vi "Centauro Verify Display Dryer.vi"(0 "GEA2 Reference In":refnum<k24>, 1 "Service Mode?":bool, 5 "UI GEA Inputs":T3={"Source"=228, "Destination"=37} {"Destination" format="%.0x"; "Source" format="%.0x"}, 7 "Care":T4={"Damp"=TRUE, "Dry"=TRUE, "Cool"=TRUE, "Eco"=TRUE}, 9 "Expected LED Status":T6, 11 "Error In":errorcluster, 12 "Erd_UiLedBitmap ERD #":T1[](array[typedef])=[{"ERD Number"=61729, "Data Type"=enum."string"}] {"ERD Number" format="%.0x"}, 13 "Erd_UiBlinkingLedBitmap ERD #":T1[](array[typedef])=[{"ERD Number"=61730, "Data Type"=enum."string"}] {"ERD Number" format="%.0x"}) -> (3 "Normal LED Binary Number Out":u32, 4 "GEA2 Reference Out":refnum<k24>, 6 "Pass/Fail?":bool, 8 "Report Text":string, 14 "Blinking LED Binary Number Out":u32, 15 "Error Out":errorcluster)   [LabVIEW 2016]
uses:
  Q:/Common/DLLs/GEA3/GeaCommunication.dll
  Common/DLLs/GEA3/GeaCommunication.dll
  Centauro Washer/Product Testcode/Centauro/Valew Common/type defs/LED Status OOB.ctl
  Common/LabVIEW GEA2 Toolkit/LabVIEW_GEA2_Toolkit.lvlibp/type defs/Source_Destination.ctl
  Common/LabVIEW GEA2 Toolkit/LabVIEW_GEA2_Toolkit.lvlibp/type defs/ERD Read Data In.ctl
  Common/LabVIEW GEA2 Toolkit/LabVIEW_GEA2_Toolkit.lvlibp/type defs/Data Type.ctl
  Common/LabVIEW GEA2 Toolkit/LabVIEW_GEA2_Toolkit.lvlibp
panel:
  in  "Board Index":i32
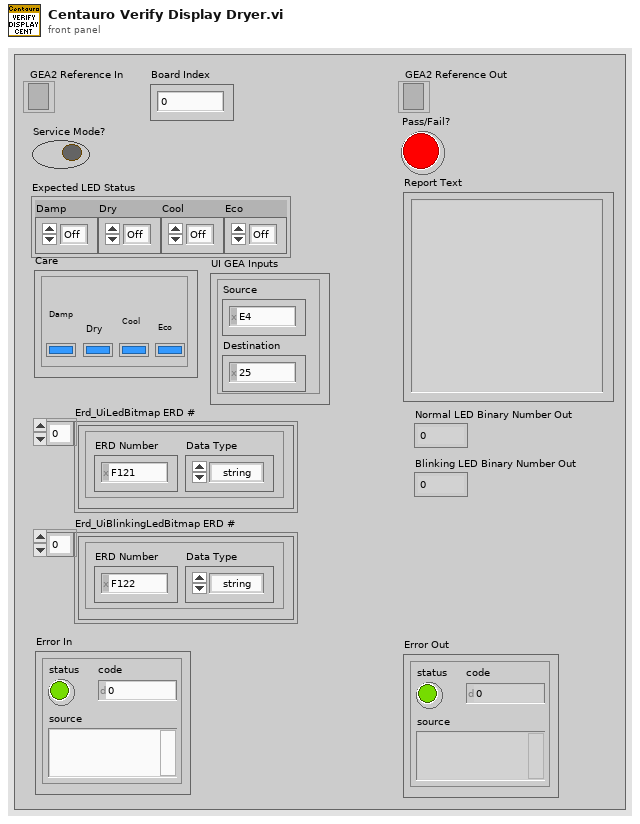
[diagram p1: front panel]
types:
  T1 = typedef "LabVIEW_GEA2_Toolkit.lvlibp/ERD Read Data In.ctl" = cluster{"ERD Number":u16, "Data Type":T2}
  T2 = typedef "LabVIEW_GEA2_Toolkit.lvlibp/Data Type.ctl" = enum16{"string", "boolean", "uint8_t", "uint16_t", "uint32_t", "uint64_t", "int8_t", "int16_t", "int32_t", "int64_t"}
  T3 = typedef "LabVIEW_GEA2_Toolkit.lvlibp/Source_Destination.ctl" = cluster{"Source":u8, "Destination":u8}
  T4 = cluster{"Damp":bool, "Dry":bool, "Cool":bool, "Eco":bool}
  T5 = typedef "LED Status OOB.ctl" = enum32{"Off", "On", "Blink"}
  T6 = cluster{"Damp":T5, "Dry":T5, "Cool":T5, "Eco":T5}
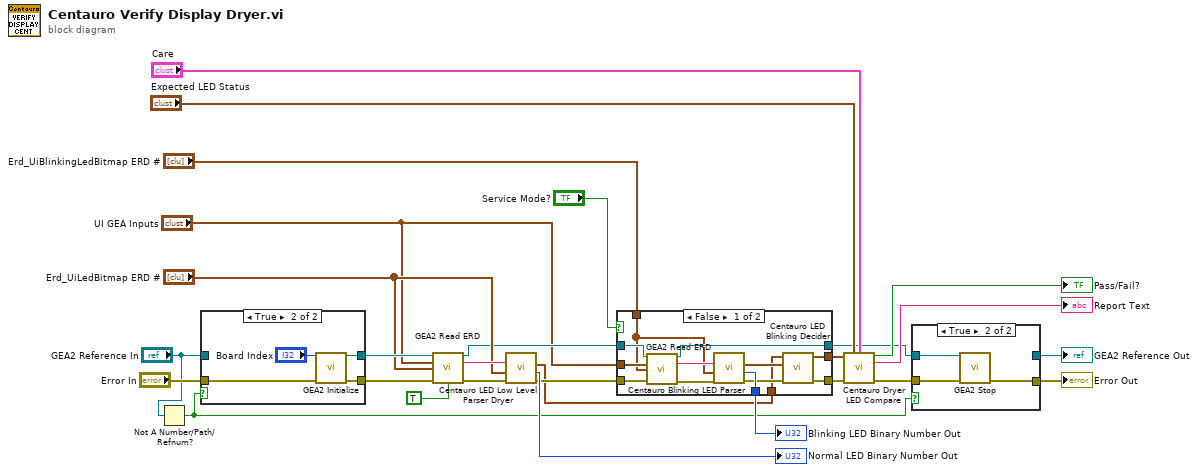
[diagram p0: block diagram]
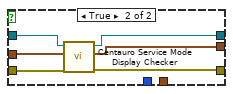
[diagram p2: hidden frame]
diagram:
  n1 = Not A Number/Path/Refnum?(number/path/refnum="GEA2 Reference In") -> (NaN/Path/Refnum?=w2:bool)
  n2 = case shown="True" w2 {
    tunnel: [w28 w33] -> w26
    tunnel: "Error In" -> [w28 w32]
    tunnel: [w29 w31] -> w24
    tunnel: "GEA2 Reference In" -> [w29 _]
    frame False {
    }
    frame True {
      n3 = call "GEA2 Initialize.vi"("Board Index"="Board Index", "error in"=w32) -> ("GEA2 Reference Out"=w31:refnum<k24>, "error out"=w33:errorcluster)  [unwired: 11 in, 1 out]
    }
  }
  n4 = call "GEA2 Read ERD.vi"("GEA2 Reference In"=w24, "GEA Inputs"="UI GEA Inputs", "Read ERD List"="Erd_UiLedBitmap ERD #", "Error In"=w26, "Verify ERD Response?"=TRUE) -> ("GEA2 Reference Out"=w12:refnum<k24>, "Raw Data Out"=w21:string, "Error Out"=w16:errorcluster)  [unwired: 7 in, 1 out]
  n5 = call "Centauro LED Low Level Parser Dryer.vi"("error in (no error)"=w16, "Read ERD List"="Erd_UiLedBitmap ERD #", "Raw Data In"=w21) -> ("error out"=w10:errorcluster, "Binary Number"=→"Normal LED Binary Number Out":u32, "LED Status"=w6:T6)  [unwired: 6 in]
  n6 = case shown="False" "Service Mode?" {
    tunnel: w12 -> [w46 w49]
    tunnel: [w45 w50] -> w11
    tunnel: w10 -> [w44 w52]
    tunnel: [w34 w51] -> w4
    tunnel: "UI GEA Inputs" -> [w42 w48]
    tunnel: "Erd_UiBlinkingLedBitmap ERD #" -> [w39 _]
    tunnel: [w40 _] -> w7
    tunnel: w6 -> [w36 _]
    tunnel: [w35 w47] -> w5
    frame False {
      n7 = call "GEA2 Read ERD.vi"("GEA2 Reference In"=w46, "GEA Inputs"=w42, "Read ERD List"=w39, "Error In"=w44) -> ("GEA2 Reference Out"=w45:refnum<k24>, "Raw Data Out"=w41:string, "Error Out"=w43:errorcluster)  [unwired: 8 in, 1 out]
      n8 = call "Centauro Blinking LED Parser.vi"("error in (no error)"=w43, "Read ERD List"=w39, "Raw Data In"=w41) -> ("error out"=w38:errorcluster, "Blinking LED Binary Number"=w40:u32, "LED Status"=w37:T6)  [unwired: 6 in]
      n9 = call "Centauro LED Blinking Decider.vi"("Error In"=w38, "Blinking LED Status"=w37, "Normal LED Status"=w36) -> ("Error Out"=w34:errorcluster, "Final LED Status"=w35:T6)  [unwired: 7 in]
    }
    frame True {
      n10 = call "Centauro Service Mode Display Checker.vi"("Error In"=w52, "UI GEA Inputs"=w48, "GEA2 Reference In"=w49) -> ("Error Out"=w51:errorcluster, "LED Status Out"=w47:T6, "GEA2 Reference Out"=w50:refnum<k24>)  [unwired: 5 in, 1 out]
    }
  }
  "Blinking LED Binary Number Out" <- w7
  n11 = call "Centauro Dryer LED Compare.vi"("Actul LED Status"=w5, "Expected LED Status"="Expected LED Status", "Care"="Care", "Error In"=w4) -> ("Pass/Fail?"=→"Pass/Fail?":bool, "Report Text"=→"Report Text":string, "Error Out"=w17:errorcluster)  [unwired: 9 in]
  n12 = case shown="True" w2 {
    tunnel: [w53 w57] -> w23
    tunnel: [w54 _] -> w22
    tunnel: w11 -> [w54 w56]
    tunnel: w17 -> [w53 w55]
    frame False {
    }
    frame True {
      n13 = call "GEA2 Stop.vi"("GEA2 Reference In"=w56, "Error In"=w55) -> ("Error Out"=w57:errorcluster)  [unwired: 13 in]
    }
  }
  "GEA2 Reference Out" <- w22
  "Error Out" <- w23
